vi "EventDrivenPluginDemo.vi"() -> ()   [LabVIEW 2017]
doc: "Use this template to build a user interface event handler design pattern. Use this pattern for dialog boxes and other user interfaces. You also can create and execute user-defined events that the VI can handle the same way as user interface events."
uses:
  EventHandler/SystemEventData/ResultType.ctl
  EventHandler/SystemEventData/EnableChangeEventData.ctl
  EventHandler/SystemEventData/ResultEventData.ctl
  EventHandler/SystemEventData/TriggerEventData.ctl
  EventHandler/SystemEventData/InfoEventData.ctl
  EventHandler/ActionsOnEvent_class/ActionsOnEvents.lvclass
  EventHandler/SystemEvents/SystemEvents_class/SystemEvents.lvclass
panel:
  in  "SystemInfo":string
  in  "IniFile":path
  in  "ActionsClass":string(combo)
  in  "Launch":bool
  in  "Result 2":T1
  in  "DeviceID":string="DemoDevice"
  in  "State":bool
  in  "Result":bool
  out "Boolean":bool
  in  "Measured":dbl(slide)=3.2335329341317367 scale=0.0..10.0
  in  "Trigger":dbl(slide)=4.491017964071856 scale=0.0..10.0
  out "Waveform Chart":cluster{"Value":dbl, "Trigger":dbl}(graph)={"Value"=3.2335329341317367, "Trigger"=4.491017964071856}
  in  "Enable":bool
  in  "stop":bool
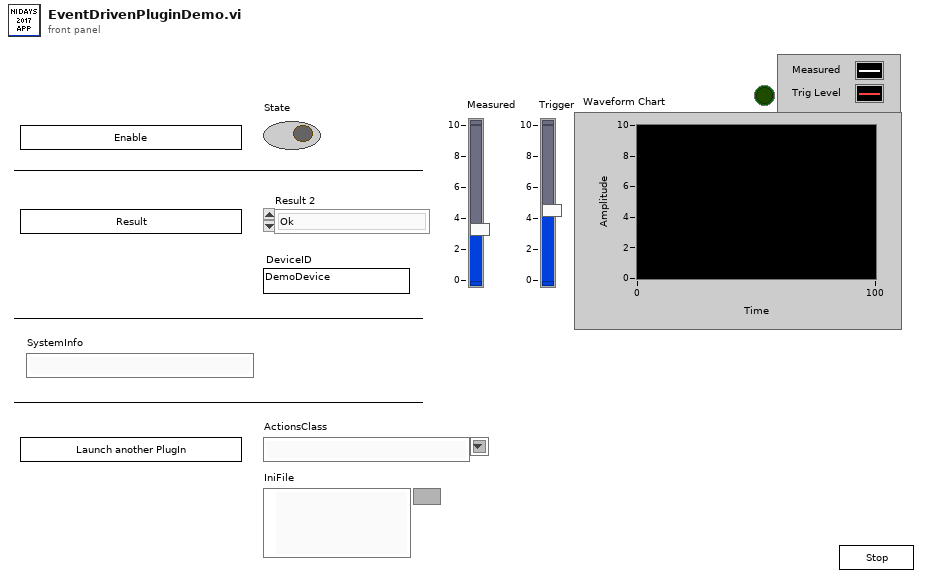
[diagram p1: front panel]
types:
  T1 = typedef "ResultType.ctl" = enum16{"Ok", "Outside limits", "Bad reading", "CtrlMeas OK", "CtrlMeas Not OK"}
  T2 = typedef "EnableChangeEventData.ctl" = cluster{"State":bool, "Registered PUT":string}
  T3 = typedef "ResultEventData.ctl" = cluster{"DeviceID":string, "RegisteredPUT":string, "TrigTime":timestamp, "Result":T1, "MeasuredValue(mg/L)":dbl}
  T4 = typedef "TriggerEventData.ctl" = cluster{"TriggerTime":timestamp, "PUT Info":string, "DeviceID":string}
  T5 = typedef "InfoEventData.ctl" = cluster{"Info":string}
  T6 = typedef "SystemEventsType.ctl" = cluster{"TrigOn":refnum<user-event>, "TrigOff":refnum<user-event>, "Result":refnum<user-event>, "Enable":refnum<user-event>, "Stop":refnum<user-event>, "AnalysisCompleted":refnum<user-event>, "Info":refnum<user-event>}
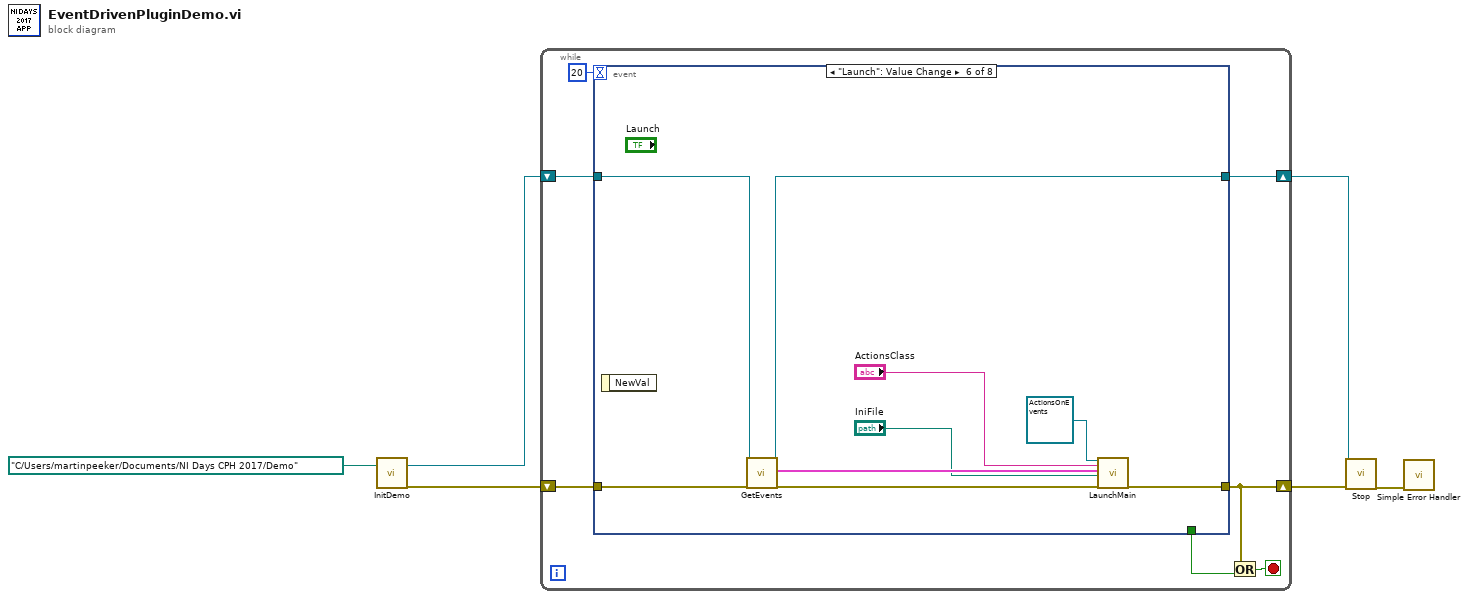
[diagram p0: block diagram]
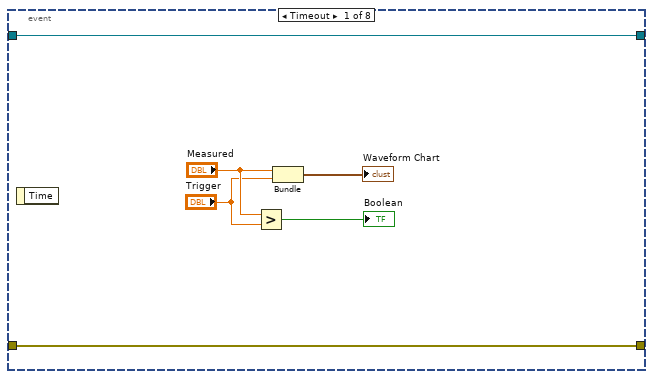
[diagram p2: hidden frame]
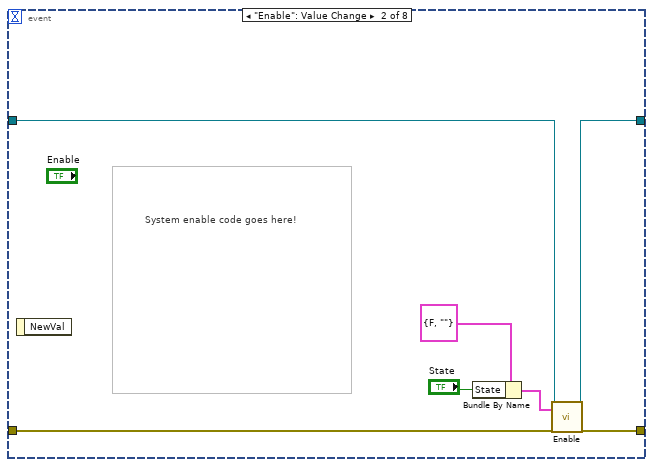
[diagram p3: hidden frame]
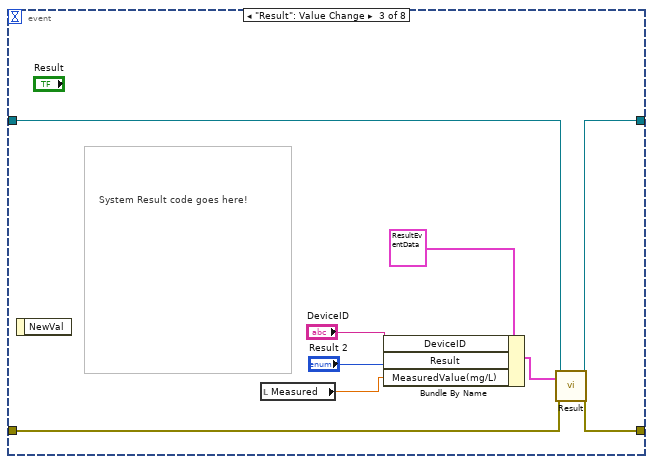
[diagram p4: hidden frame]
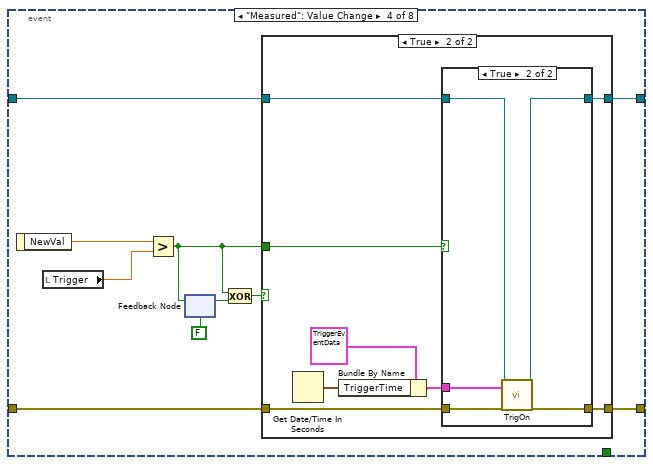
[diagram p5: hidden frame]
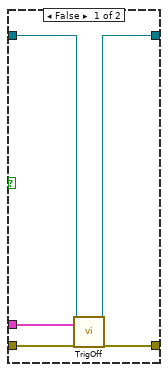
[diagram p7: hidden frame]
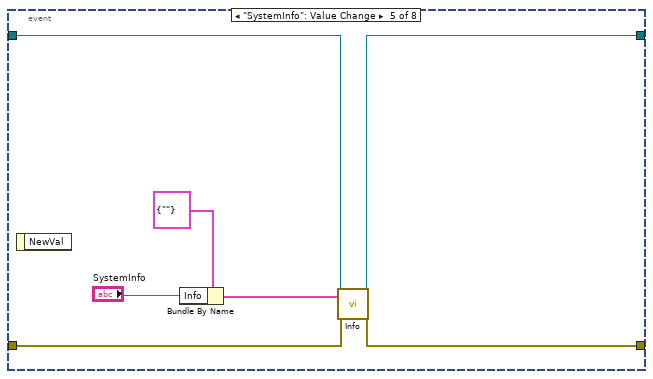
[diagram p8: hidden frame]
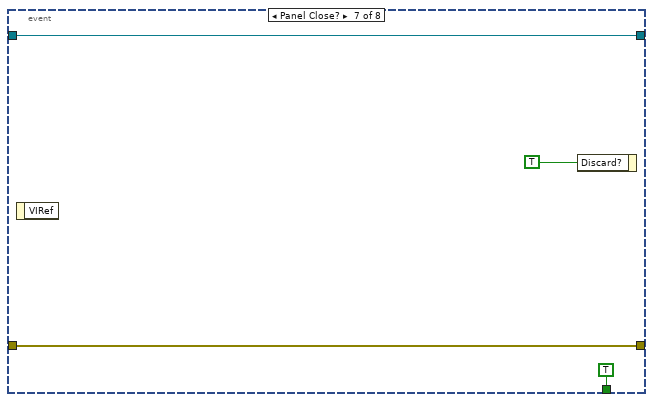
[diagram p9: hidden frame]
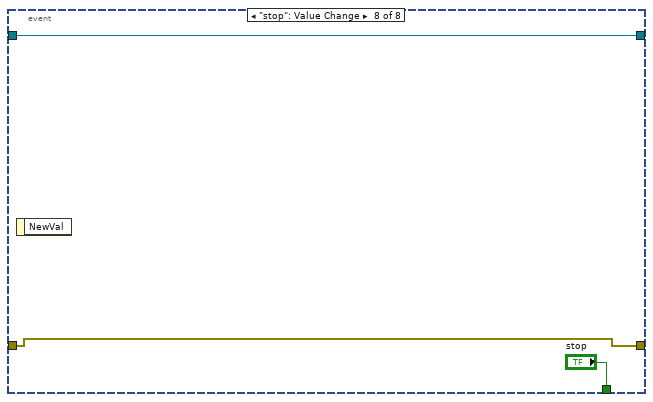
[diagram p10: hidden frame]
diagram:
  n1 = call "InitDemo.vi"("IniFileDir"=path "C:/Users/martinpeeker/Documents/NI Days CPH 2017/Demo") -> ("SystemEvents.lvclass out"=w2:refnum<class "SystemEvents.lvclass">, "error out"=w4:errorcluster)  [unwired: 17 in]
  n2 = while {
    shift-right: [w9] -> w6
    shift-left: w4 -> [w11]
    shift-right: [w7] -> w1
    shift-left: w2 -> [w8]
    stop <- w10 stop-if-true
    n3 = event shown="[5] \"Launch\": Value Change" {
      selector: _ -> [_ _ _ _ _ _ _ _]
      dyn-events: _ -> [_ _ _ _ _ _ _ _]
      timeout: 20 -> [_ _ _ _ _ _ _ _]
      tunnel: [_ _ _ _ _ _ TRUE ("stop") "stop"] -> w13
      tunnel: w11 -> [w15 w26 w35 w43 w69 w78 w85 w87]
      tunnel: [w15 w25 w34 w42 w68 w73 w85 w87] -> w9
      tunnel: [w14 w20 w28 w36 w66 w76 w82 w86] -> w7
      tunnel: w8 -> [w14 w21 w29 w37 w67 w77 w82 w86]
      event Timeout {
        n4 = event-data() -> ()  [unwired: 1 in, 1 out]
        n5 = Greater?(x="Measured", y="Trigger") -> (0:→"Boolean":bool)
        n6 = Bundle("Measured"="Measured", "Trigger"="Trigger") -> (→"Waveform Chart":cluster{"Measured":dbl, "Trigger":dbl})  [unwired: 1 in]
      }
      event "Enable": Value Change {
        # "System enable code goes here!"
        n7 = event-data() -> ()  [unwired: 1 in, 1 out]
        n8 = Bundle By Name(cluster=T2 {"State"=FALSE, "Registered PUT"=""} ("event data"), "State"="State") -> (w22:T2)
        n9 = call-dynamic "Enable.vi"("SystemEvents in"=w21, "event data"=w22, "error in (no error)"=w26) -> ("SystemEvents out"=w20:refnum<class "SystemEvents.lvclass">, "error out"=w25:errorcluster)  [unwired: 15 in]
      }
      event "Result": Value Change {
        # "System Result code goes here!"
        n10 = event-data() -> ()  [unwired: 1 in, 1 out]
        n11 = local read "Measured"() -> (w27:dbl)
        n12 = Bundle By Name(cluster=T3 {"DeviceID"="", "RegisteredPUT"="", "TrigTime"=timestamp(0 s since 1904-01-01), "Result"=enum."Ok", "MeasuredValue(mg/L)"=0.0} ("event data"), "DeviceID"="DeviceID", "Result"="Result 2", "MeasuredValue(mg/L)"=w27) -> (w30:T3)
        n13 = call-dynamic "Result.vi"("SystemEvents in"=w29, "event data"=w30, "error in (no error)"=w35) -> ("SystemEvents out"=w28:refnum<class "SystemEvents.lvclass">, "error out"=w34:errorcluster)  [unwired: 15 in]
      }
      event "Measured": Value Change {
        n14 = event-data() -> ("NewVal"=w44:dbl)  [unwired: 1 in]
        n15 = local read "Trigger"() -> (w45:dbl)
        n16 = Greater?(x=w44, y=w45) -> (0:w40:bool)
        n17 = feedback-in #1(w40) -> ()
        n18 = feedback #1(FALSE) -> (w39:bool)
        n19 = Exclusive Or(1:w39, 2:w40) -> (0:w41:bool)
        n20 = case shown="True" w41 {
          tunnel: w43 -> [w47 w54]
          tunnel: w40 -> [_ w55]
          tunnel: [w47 w53] -> w42
          tunnel: w37 -> [w46 w49]
          tunnel: [w46 w48] -> w36
          frame False {
          }
          frame True {
            n21 = Get Date/Time In Seconds() -> (seconds since 1Jan1904=w51:timestamp)
            n22 = Bundle By Name(cluster=T4 {"TriggerTime"=timestamp(0 s since 1904-01-01), "PUT Info"="", "DeviceID"="DemoDevice"} ("event data"), "TriggerTime"=w51) -> (w50:T4)
            n23 = case shown="True" w55 {
              tunnel: w54 -> [w60 w65]
              tunnel: [w59 w64] -> w53
              tunnel: w50 -> [w58 w63]
              tunnel: w49 -> [w57 w62]
              tunnel: [w56 w61] -> w48
              frame False {
                n24 = call-dynamic "TrigOff.vi"("SystemEvents in"=w57, "event data"=w58, "error in (no error)"=w60) -> ("SystemEvents out"=w56:refnum<class "SystemEvents.lvclass">, "error out"=w59:errorcluster)  [unwired: 15 in]
              }
              frame True {
                n25 = call-dynamic "TrigOn.vi"("SystemEvents in"=w62, "event data"=w63, "error in (no error)"=w65) -> ("SystemEvents out"=w61:refnum<class "SystemEvents.lvclass">, "error out"=w64:errorcluster)  [unwired: 15 in]
              }
            }
          }
        }
      }
      event "SystemInfo": Value Change {
        n26 = event-data() -> ()  [unwired: 1 in, 1 out]
        n27 = Bundle By Name(cluster=T5 {"Info"=""} ("InfoEventData"), "Info"="SystemInfo") -> (w70:T5)
        n28 = call-dynamic "Info.vi"("SystemEvents in"=w67, "event data"=w70, "error in (no error)"=w69) -> ("SystemEvents out"=w66:refnum<class "SystemEvents.lvclass">, "error out"=w68:errorcluster)  [unwired: 15 in]
      }
      event "Launch": Value Change {
        n29 = event-data() -> ()  [unwired: 1 in, 1 out]
        n30 = call-dynamic "GetEvents.vi"("SystemEvents.lvclass in"=w77, "error in (no error)"=w78) -> ("SystemEvents.lvclass out"=w76:refnum<class "SystemEvents.lvclass">, "Events"=w80:T6, "error out"=w79:errorcluster)  [unwired: 15 out]
        n31 = call "LaunchMain.vi"("ActionsOnEvents in"=refnum<class "ActionsOnEvents.lvclass"> refnum, "ActionsClass"="ActionsClass", "Events"=w80, "IniFile"="IniFile", "error in (no error)"=w79) -> ("error out"=w73:errorcluster)  [unwired: 14 out]
      }
      event Panel Close? {
        n32 = event-data() -> ()  [unwired: 1 in, 1 out]
        n33 = event-data("Discard?"=TRUE) -> ()  [unwired: 1 in, 1 out]
      }
      event "stop": Value Change {
        n34 = event-data() -> ()  [unwired: 1 in, 1 out]
      }
    }
    n35 = Or(x=w9, y=w13) -> (x .or. y?=w10:bool)
  }
  n36 = call-dynamic "Stop.vi"("SystemEvents in"=w1, "error in (no error)"=w6) -> ("error out"=w5:errorcluster)  [unwired: 16 in, 1 out]
  n37 = call <vilib>:"Simple Error Handler.vi"("error in (no error)"=w5) -> ()  [unwired: 4 in, 5 out]
